vi "Dequeue Message.vi"(6 "timeout in ms (-1)":i32, 8 "error in (no error)":errorcluster, 11 "Queue In":T1) -> (0 "error out":errorcluster, 1 "Data":variant, 2 "Command":string, 3 "Queue Out":T1)   [LabVIEW 2023, in "Innes Process Communication.lvlib"]
doc: "Dequeue Message from selected Inner Process Queue"
uses:
  Innes Process Communication.lvlib
  Queue Type Reference.ctl
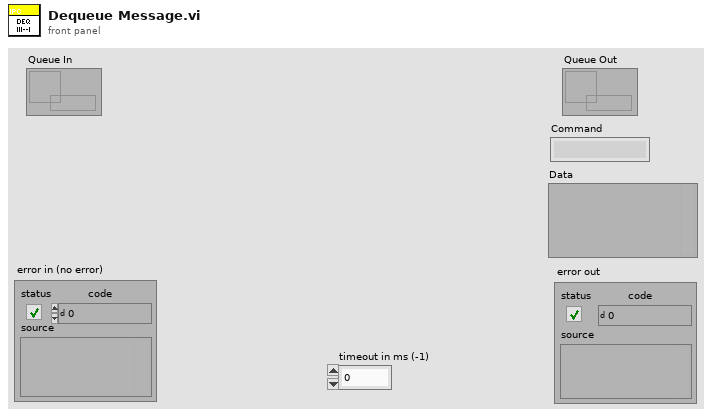
[diagram p1: front panel]
types:
  T1 = typedef "Innes Process Communication.lvlib/Queue Type Reference.ctl" = refnum<queue>
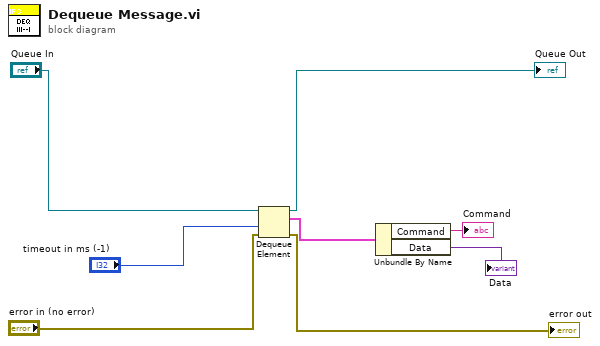
[diagram p0: block diagram]
diagram:
  n1 = Dequeue Element(queue="Queue In", timeout in ms (-1)="timeout in ms (-1)", error in (no error)="error in (no error)") -> (queue out=→"Queue Out":T1, element=w4:cluster{"Command":string, "Data":variant}, error out=→"error out":errorcluster)  [unwired: 1 out]
  n2 = Unbundle By Name(w4) -> ("Command"=→"Command":string, "Data"=→"Data":variant)
